vi "Remove Item.vi"(8 "error in (no error)":errorcluster, 10 "Item Configuration":T1, 11 "Assert Display in":refnum<class "Assert Display.lvclass">) -> (0 "error out":errorcluster, 3 "Assert Display out":refnum<class "Assert Display.lvclass">)   [LabVIEW 2016, in "Assert API Components.lvlib" / "Assert Display.lvlib" / "Assert Display.lvclass"]
uses:
  Assert Display.lvclass
  Item Configuration.ctl
  Service Config Display/Service Config Display/Items.ctl
  Assert Display.lvclass/Assert Display.ctl
  Main Display/Main Display Messages/Remove Named Filter Msg/Remove Named Filter Msg.lvclass/Remove Named Filter Msg.ctl
  <vilib>/ActorFramework/Message Enqueuer/Message Enqueuer.lvclass/Message Enqueuer.ctl
  <vilib>/ActorFramework/Message Enqueuer/Enqueue.vi
  Main Display/Main Display Messages/Remove Named Filter Msg/Remove Named Filter Msg.lvclass
  C:/Program Files (x86)/National Instruments/LabVIEW 2016/vi.lib/ActorFramework/Message/Message.lvclass
  <vilib>/Utility/LVClass/Get LV Class Name.vi
  <resource>/AFDebug/Generate Trace for Message.vi
  <vilib>/ActorFramework/Message Priority Queue/Priority Enqueue.vi
  Assert Display.lvlib
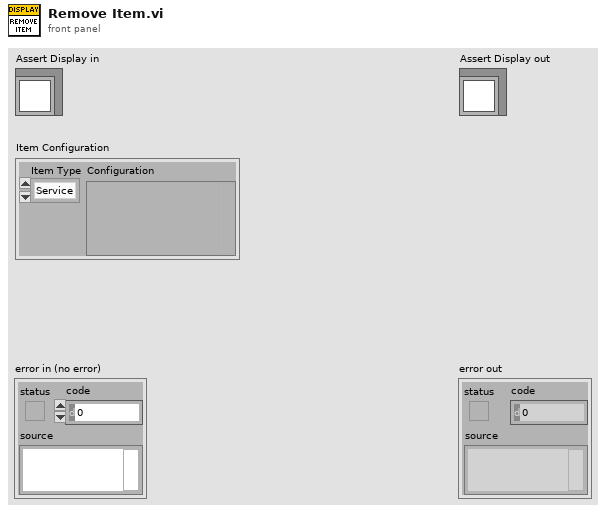
[diagram p1: front panel]
types:
  T1 = typedef "Assert API Components.lvlib/Assert Display.lvlib/Item Configuration.ctl" = cluster{"Item Type":T2, "Configuration":variant}
  T2 = typedef "Assert API Components.lvlib/Assert Display.lvlib/Items.ctl" = enum16{"Service", "Filter"}
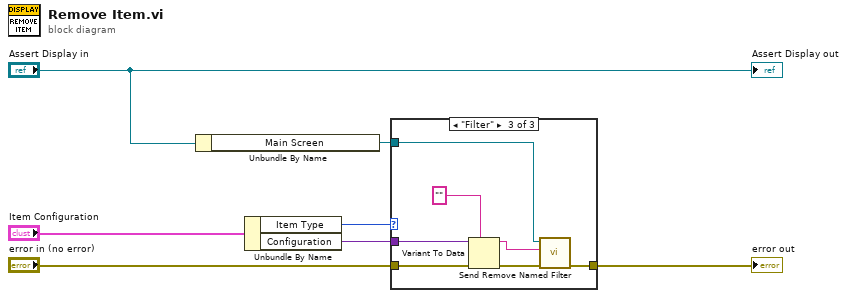
[diagram p0: block diagram]
diagram:
  n1 = Unbundle By Name("Assert Display in") -> ("Main Screen"=w5:refnum<class "Message Enqueuer.lvclass">)
  n2 = Unbundle By Name("Item Configuration") -> ("Item Type"=w7:T2, "Configuration"=w6:variant)
  n3 = case shown="\"Filter\"" w7 {
    tunnel: w6 -> [_ _ w13]
    tunnel: w5 -> [_ _ w11]
    tunnel: "error in (no error)" -> [w8 w9 w16]
    tunnel: [w8 w9 w15] -> w1
    frame "Service" {
    }
    frame Default {
    }
    frame "Filter" {
      n4 = Variant To Data(error in=w16, type="" ("New Filter"), Variant=w13) -> (data=w10:string, error out=w14:errorcluster)
      n5 = call "Send Remove Named Filter.vi"("error in (no error)"=w14, "Filter Name"=w10, "Message Enqueuer"=w11) -> ("error out"=w15:errorcluster)  [unwired: 7 in, 1 out]
    }
  }
  "error out" <- w1
  "Assert Display out" <- "Assert Display in"
